vi "RunAllTests.vi"() -> ()   [LabVIEW 2019]
uses:
  <vilib>/Rock Robotics/WPI/ThirdParty/JAS_Junk/TrajLib/Trajectory_Library.lvlib
panel:
  out "Meca Drive \nPose Est 2":bool
  out "Swerve Module Position":bool
  out "Swerve Drive Pose Est 2":bool
  out "Diff Drive Pose Est 2":bool
  out "Diff Drive Odom 2":bool
  out "April Tag":bool
  out "Vector":bool
  out "Lead Lag":bool
  out "Elliptical Region\nConstraint":bool
  out "Rectangular Region\nConstraint":bool
  out "Meca Drive \nPose Est":bool
  out "Coordinate System":bool
  out "Meca Drive \nOdometry":bool
  out "Meca Drive \nKinematics":bool
  out "Pose3d":bool
  out "Transform3d":bool
  out "Rotation3d":bool
  out "Translation3d":bool
  out "Twist3d":bool
  out "Function Generator \nMatrix":bool
  out "LTV Unicycle \nController":bool
  out "LTV Diff Drive \nController":bool
  out "Time Interpolatable \nRotation2d":bool
  out "Time Interpolatable \nDouble":bool
  out "Time Interpolatable \nBoolean":bool
  out "Time Interpolatable \nPose2d":bool
  out "Implicit Model \nFollower":bool
  out "Function Generator":bool
  out "Diff Drive Accel Limiter":bool
  out "String":string
  out "Vision Utilities":bool
  out "Flywheel Simulation":bool
  out "DC Motor Simulation":bool
  out "Matrix":bool
  out "PID":bool
  out "Profiled PID \nInput/Output":bool
  out "Bang Bang \nInput/Output":bool
  out "Bang Bang Tolerance":bool
  out "Debounce":bool
  out "Math Utils":bool
  out "Linear Filter":bool
  out "State Space Util":bool
  out "Runge Kutta \nTime Varying":bool
  out "Linear System Loop":bool
  out "Swerve Drive \nKinematics":bool
  out "Swerve Drive Odometry":bool
  out "Trajectory Generate":bool
  out "Trajectory Transform":bool
  out "Units":bool
  out "All Tests Finished":bool
  out "Trajectory Concatenate":bool
  out "Trajectory JSON":bool
  out "Diff Drive Train Sim":bool
  out "Timer":bool
  out "Single Jointed \nArm Sim":bool
  out "Elevator Sim":bool
  out "Simple Motor \nFeedforward":bool
  out "Diff Drive Voltage \nConstraint":bool
  out "Diff Drive Pose Est":bool
  out "Holonomic Drive Ctrl":bool
  out "Linear Plant Inv FF":bool
  out "Centrip Accel \nConstraint":bool
  out "Diff Drive Kine \nConstraint":bool
  out "Controller Utility":bool
  out "Swerve Drive Pose Est":bool
  out "Swerve Module State":bool
  out "Trapezoid Profile":bool
  out "Slew Rate Limiter":bool
  out "Chassis Speeds":bool
  out "Numerical Jacobian":bool
  out "Merwe Scaled \nSigma Pts":bool
  out "Numerical Integration":bool
  out "DARE - Ricatti":bool
  out "Quintic Spline":bool
  out "Unscented Kalman \nFilter":bool
  out "Ramsete":bool
  out "Profiled PID":bool
  out "Twist":bool
  out "Translation2d":bool
  out "Transform2d":bool
  out "Rotation2d":bool
  out "Pose2d":bool
  out "Median Filter":bool
  out "Cubic Spline":bool
  out "Linear System ID":bool
  out "Kalman filter":bool
  out "Discretization":bool
  out "PID tolerance":bool
  out "PID Input / Output":bool
  out "Linear Quadradtic \nRegulator":bool
  out "Diff Drive Kinematics":bool
  out "Angle Stats":bool
  # "FORMAL TRAJECTORY / CONTROL LIBRARY TEST PROCEDURE"
  # "FUNCTION NOT\nIMPLEMENTED"
  # "Extended Kalman \nFilter"
  # "Cntrl Affine Plant \nInversion"
  # "FUNCTION NOT\nIMPLEMENTED"
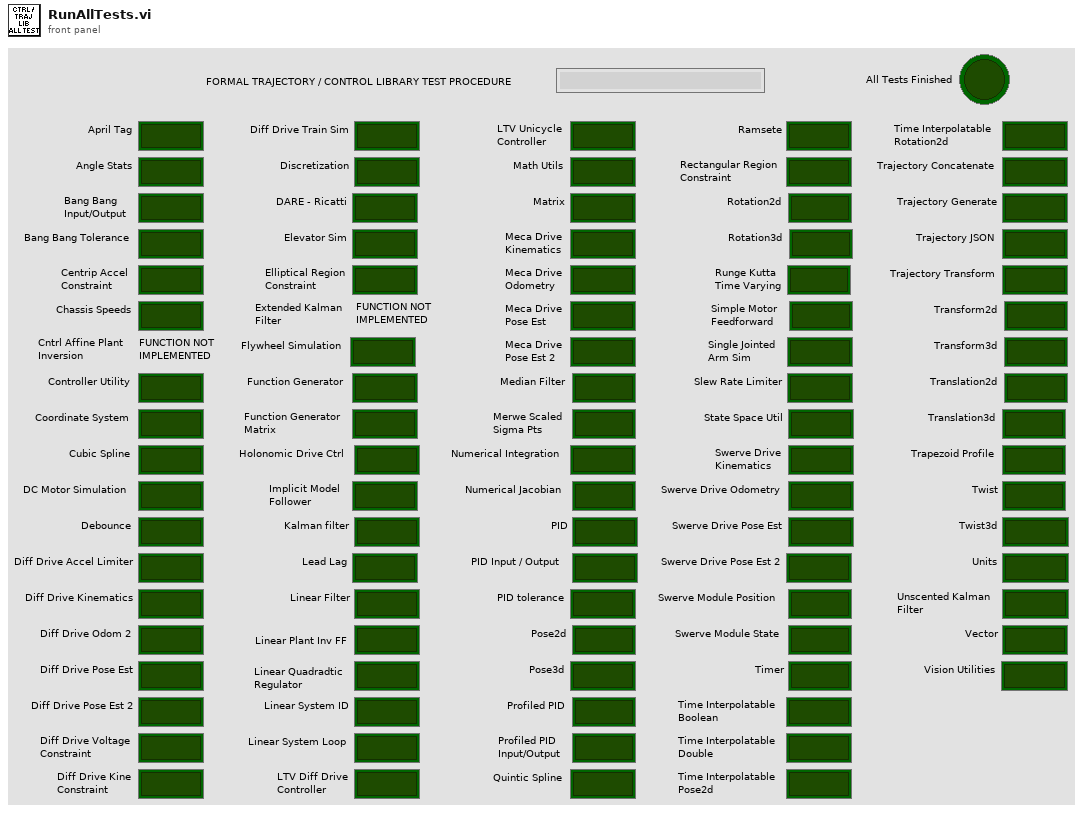
[diagram p1: front panel]
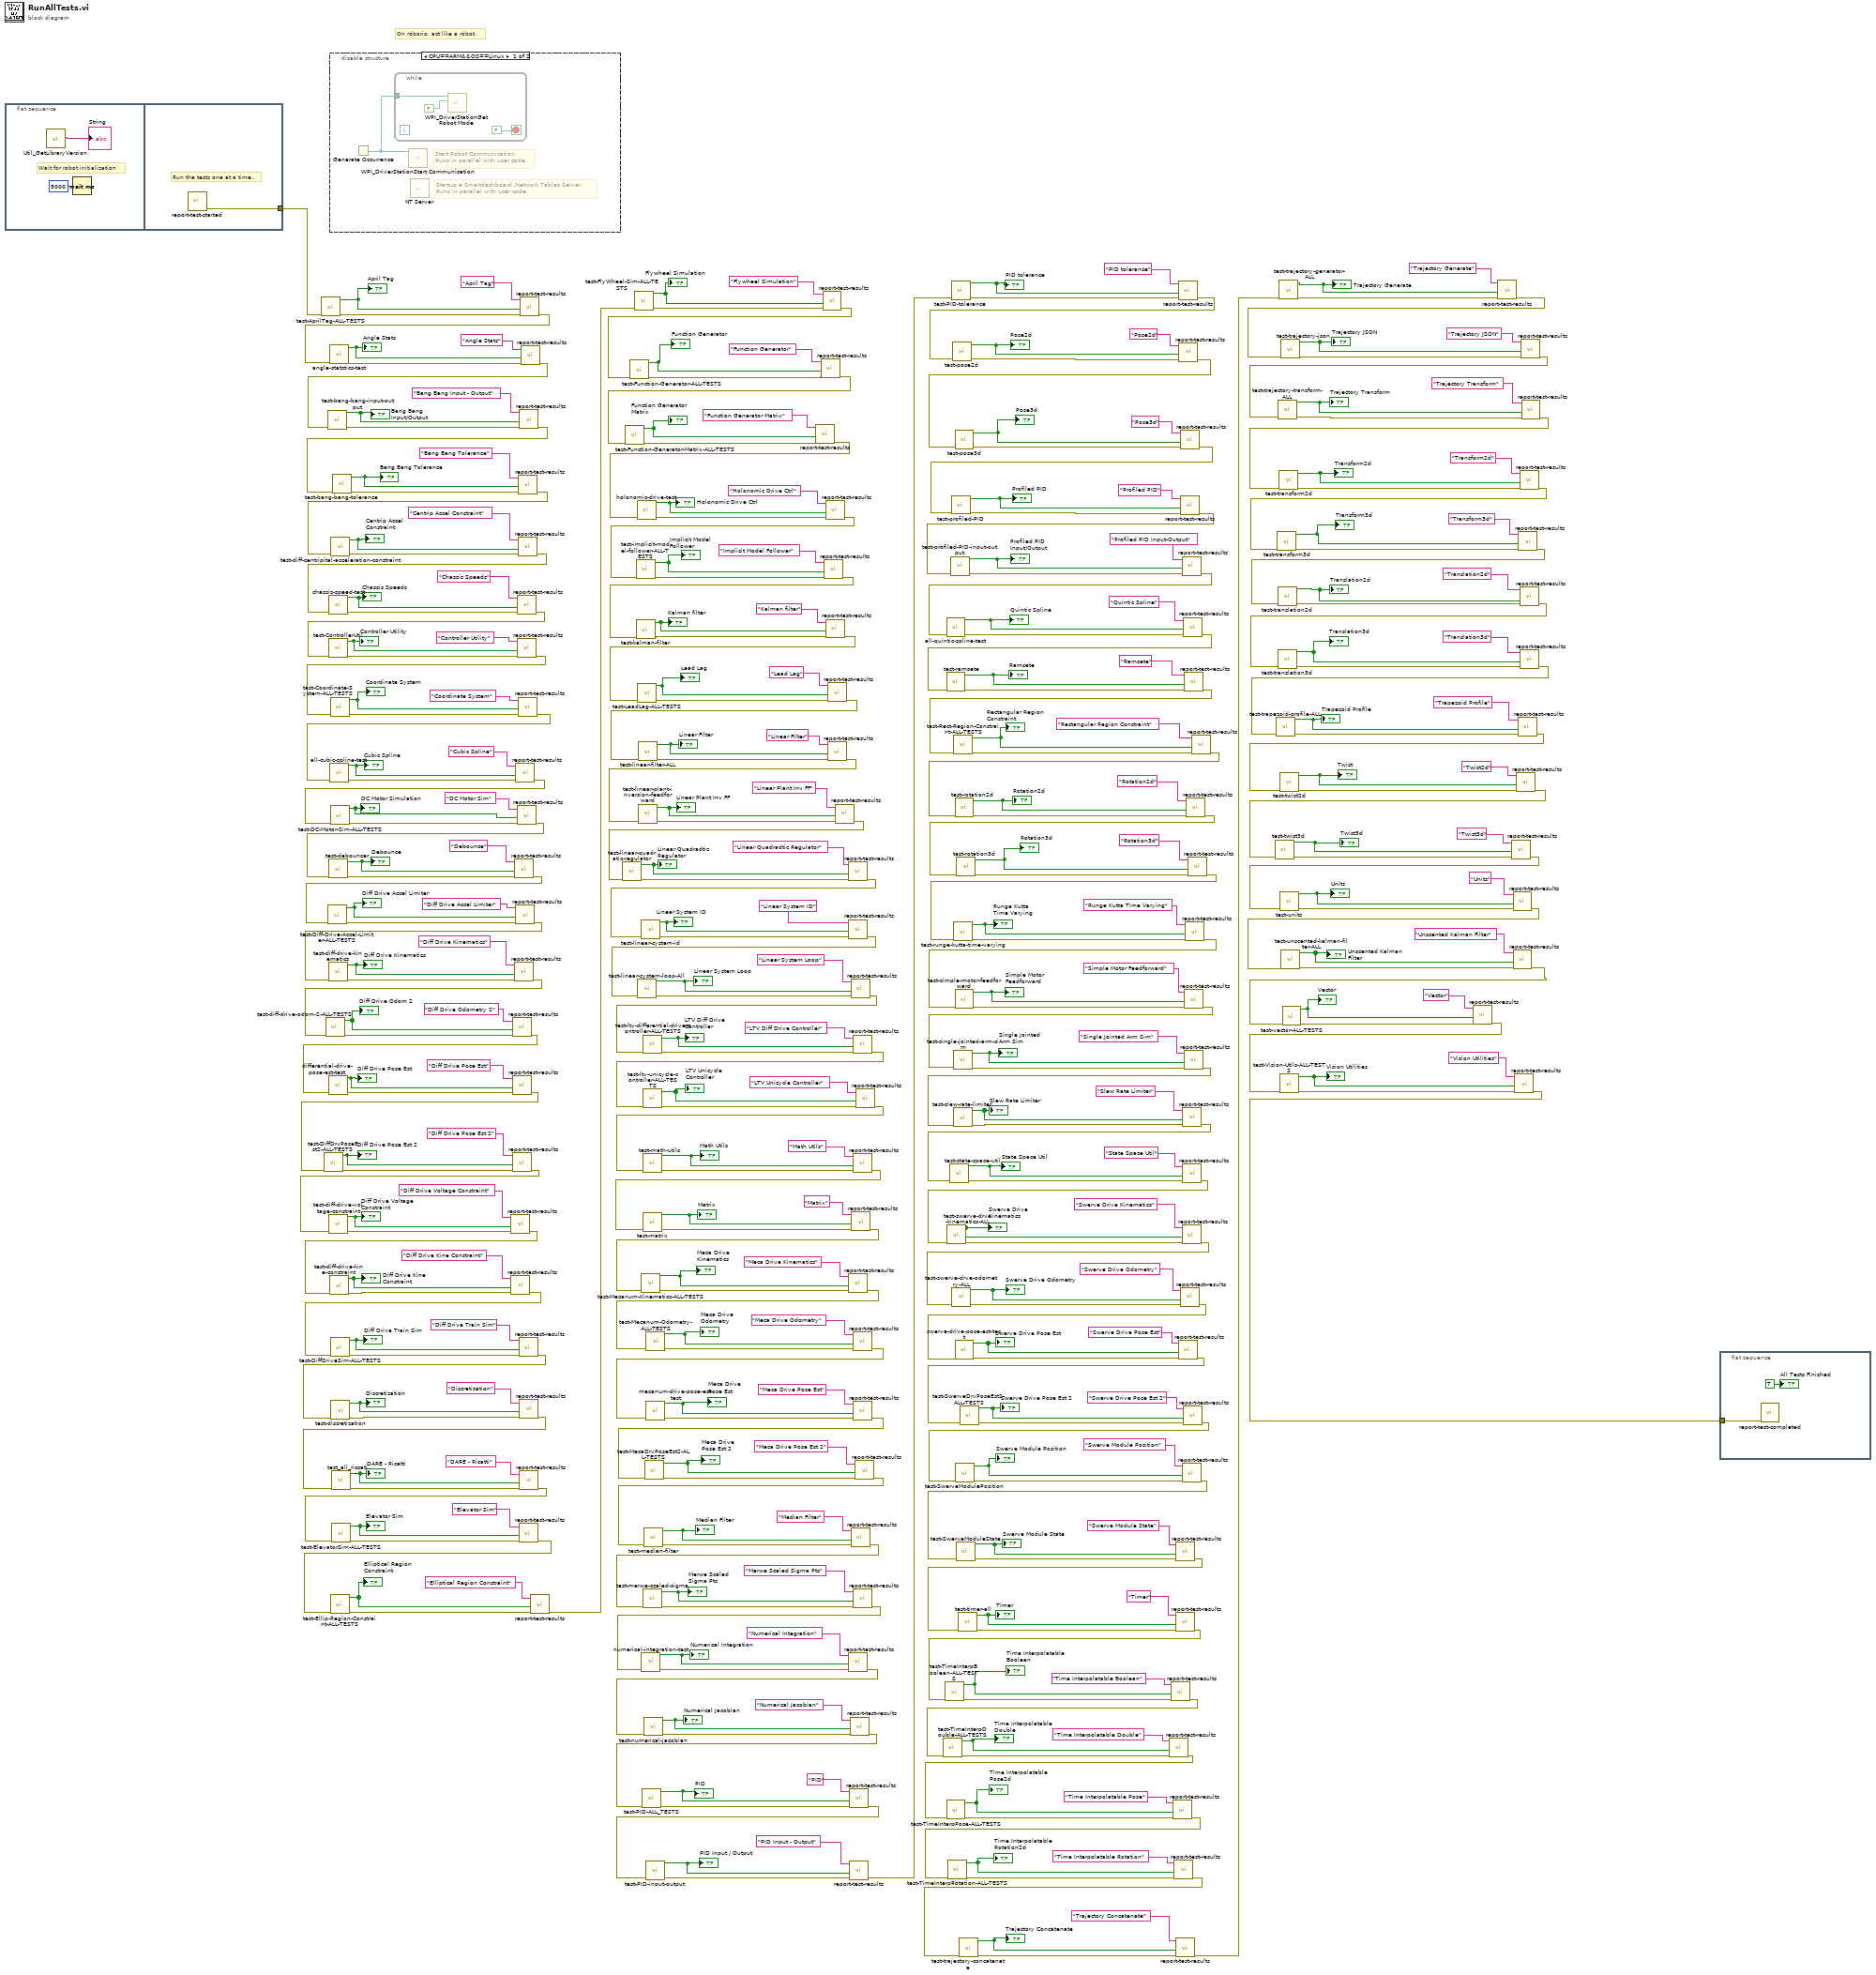
[diagram p0: block diagram]
diagram:
  # "On roborio, act like a robot."
  n1 = flat-sequence {
    tunnel: [w364] -> w16
    frame #0 {
      # "Wait for robot initialization"
      n2 = call <vilib>:"Util_GetLibraryVersion.vi"() -> ("TrajLibVersion"=→"String":string)  [unwired: 11 in]
      n3 = Wait (ms)(milliseconds to wait=u32 5000) -> ()  [unwired: 1 out]
    }
    frame #1 {
      # "Run the tests one at a time.."
      n4 = call "report-test-started.vi"() -> ("error out"=w364:errorcluster)  [unwired: 11 in]
    }
  }
  n5 = call "test-AprilTag-ALL-TESTS.vi"("error in (no error)"=w16) -> ("error out"=w29:errorcluster, "All Passed"=w28:bool)  [unwired: 9 in]
  "April Tag" <- w28
  n6 = disable-structure shown="CPU==ARM&&OS==Linux" {
    frame condition #0 {
      # "Startup a Smartdashboard /Network Tables Server.\nRuns in parallel with user code."
      # "Start Robot Communication.\nRuns in parallel with user code."
      n7 = Generate Occurrence() -> (w365:refnum<k4>)
      n8 = while {
        tunnel: w365 -> [w368]
        stop <- FALSE stop-if-true
        n9 = call <vilib>:"WPI_DriverStationGet Robot Mode.vi"("Finish"=FALSE, "DS Occurrence"=w368) -> ()  [unwired: 10 out]
      }
      n10 = call <vilib>:"WPI_DriverStationStart Communication.vi"("occurrence"=w365) -> ()  [unwired: 2 in, 9 out]
      n11 = call <vilib>:"NT Server.vi"() -> ()  [unwired: 11 in, 1 out]
    }
    frame condition #1 (active) {
    }
  }
  n12 = call "report-test-results.vi"("error in (no error)"=w29, "TestPassed"=w28, "Test Name"="April Tag") -> ("error out"=w15:errorcluster)  [unwired: 8 in]
  n13 = call "angle-statstics-test.vi"("error in (no error)"=w15) -> ("error out"=w244:errorcluster, "All Passed"=w361:bool)  [unwired: 9 in]
  "Angle Stats" <- w361
  n14 = call "report-test-results.vi"("error in (no error)"=w244, "TestPassed"=w361, "Test Name"="Angle Stats") -> ("error out"=w245:errorcluster)  [unwired: 8 in]
  n15 = call "test-bang-bang-input-output.vi"("error in (no error)"=w245) -> ("error out"=w243:errorcluster, "All Tests Passed"=w358:bool)  [unwired: 9 in]
  "Bang Bang \nInput/Output" <- w358
  n16 = call "report-test-results.vi"("error in (no error)"=w243, "TestPassed"=w358, "Test Name"="Bang Bang Input - Output") -> ("error out"=w242:errorcluster)  [unwired: 8 in]
  n17 = call "test-bang-bang-tolerance.vi"("error in (no error)"=w242) -> ("error out"=w241:errorcluster, "All Tests Passed"=w356:bool)  [unwired: 9 in]
  "Bang Bang Tolerance" <- w356
  n18 = call "report-test-results.vi"("error in (no error)"=w241, "TestPassed"=w356, "Test Name"="Bang Bang Tolerance") -> ("error out"=w240:errorcluster)  [unwired: 8 in]
  n19 = call "test-diff-centripital-acceleration-constraint.vi"("error in (no error)"=w240) -> ("error out 2"=w239:errorcluster, "Test Passed"=w354:bool)  [unwired: 9 in]
  "Centrip Accel \nConstraint" <- w354
  n20 = call "report-test-results.vi"("error in (no error)"=w239, "TestPassed"=w354, "Test Name"="Centrip Accel Constraint") -> ("error out"=w238:errorcluster)  [unwired: 8 in]
  n21 = call "chassis-speed-test.vi"("error in (no error)"=w238) -> ("error out"=w237:errorcluster, "Test Passed"=w352:bool)  [unwired: 9 in]
  "Chassis Speeds" <- w352
  n22 = call "report-test-results.vi"("error in (no error)"=w237, "TestPassed"=w352, "Test Name"="Chassis Speeds") -> ("error out"=w139:errorcluster)  [unwired: 8 in]
  n23 = call "test-ControllerUtil.vi"("error in (no error)"=w139) -> ("error out"=w236:errorcluster, "All Tests Passed"=w350:bool)  [unwired: 9 in]
  "Controller Utility" <- w350
  n24 = call "report-test-results.vi"("error in (no error)"=w236, "TestPassed"=w350, "Test Name"="Controller Utility") -> ("error out"=w58:errorcluster)  [unwired: 8 in]
  n25 = call "test-Coordinate-System-ALL-TESTS.vi"("error in (no error)"=w58) -> ("error out"=w59:errorcluster, "All Passed"=w56:bool)  [unwired: 9 in]
  "Coordinate System" <- w56
  n26 = call "report-test-results.vi"("error in (no error)"=w59, "TestPassed"=w56, "Test Name"="Coordinate System") -> ("error out"=w57:errorcluster)  [unwired: 8 in]
  n27 = call "all-cubic-spline-test.vi"("error in (no error)"=w57) -> ("error out"=w230:errorcluster, "ALL TESTS PASSED"=w346:bool)  [unwired: 9 in]
  "Cubic Spline" <- w346
  n28 = call "report-test-results.vi"("error in (no error)"=w230, "TestPassed"=w346, "Test Name"="Cubic Spline") -> ("error out"=w150:errorcluster)  [unwired: 8 in]
  n29 = call "test-DC-Motor-Sim-ALL-TESTS.vi"("error in (no error)"=w150) -> ("error out"=w148:errorcluster, "All Passed"=w147:bool)  [unwired: 9 in]
  "DC Motor Simulation" <- w147
  n30 = call "report-test-results.vi"("error in (no error)"=w148, "TestPassed"=w147, "Test Name"="DC Motor Sim") -> ("error out"=w146:errorcluster)  [unwired: 8 in]
  n31 = call "test-debouncer.vi"("error in (no error)"=w146) -> ("error out"=w229:errorcluster, "ALL TESTS PASSED"=w345:bool)  [unwired: 9 in]
  "Debounce" <- w345
  n32 = call "report-test-results.vi"("error in (no error)"=w229, "TestPassed"=w345, "Test Name"="Debounce") -> ("error out"=w136:errorcluster)  [unwired: 8 in]
  n33 = call "test-Diff-Drive-Accel-Limiter-ALL-TESTS.vi"("error in (no error)"=w136) -> ("error out"=w137:errorcluster, "All Passed"=w135:bool)  [unwired: 9 in]
  "Diff Drive Accel Limiter" <- w135
  n34 = call "report-test-results.vi"("error in (no error)"=w137, "TestPassed"=w135, "Test Name"="Diff Drive Accel Limiter") -> ("error out"=w134:errorcluster)  [unwired: 8 in]
  n35 = call "test-diff-drive-kinematics.vi"("error in (no error)"=w134) -> ("error out"=w228:errorcluster, "All Passed"=w344:bool)  [unwired: 9 in]
  "Diff Drive Kinematics" <- w344
  n36 = call "report-test-results.vi"("error in (no error)"=w228, "TestPassed"=w344, "Test Name"="Diff Drive Kinematics") -> ("error out"=w26:errorcluster)  [unwired: 8 in]
  n37 = call "test-diff-drive-odom-2-ALL-TESTS.vi"("error in (no error)"=w26) -> ("error out"=w25:errorcluster, "All Passed"=w24:bool)  [unwired: 9 in]
  "Diff Drive Odom 2" <- w24
  n38 = call "report-test-results.vi"("error in (no error)"=w25, "TestPassed"=w24, "Test Name"="Diff Drive Odometry 2") -> ("error out"=w23:errorcluster)  [unwired: 8 in]
  n39 = call "differential-drive-pose-est-test.vi"("error in (no error)"=w23) -> ("error out"=w227:errorcluster, "Test Passed"=w340:bool)  [unwired: 9 in]
  "Diff Drive Pose Est" <- w340
  n40 = call "report-test-results.vi"("error in (no error)"=w227, "TestPassed"=w340, "Test Name"="Diff Drive Pose Est") -> ("error out"=w21:errorcluster)  [unwired: 8 in]
  n41 = call "test-DiffDrvPoseEst2-ALL-TESTS.vi"("error in (no error)"=w21) -> ("error out"=w20:errorcluster, "All Passed"=w19:bool)  [unwired: 9 in]
  "Diff Drive Pose Est 2" <- w19
  n42 = call "report-test-results.vi"("error in (no error)"=w20, "TestPassed"=w19, "Test Name"="Diff Drive Pose Est 2") -> ("error out"=w18:errorcluster)  [unwired: 8 in]
  n43 = call "test-diff-drive-voltage-constraint.vi"("error in (no error)"=w18) -> ("error out 4"=w226:errorcluster, "Test Passed"=w339:bool)  [unwired: 9 in]
  "Diff Drive Voltage \nConstraint" <- w339
  n44 = call "report-test-results.vi"("error in (no error)"=w226, "TestPassed"=w339, "Test Name"="Diff Drive Voltage Constraint") -> ("error out"=w221:errorcluster)  [unwired: 8 in]
  n45 = call "test-diff-drive-kine-constraint.vi"("error in (no error)"=w221) -> ("error out 2"=w225:errorcluster, "Test Passed"=w338:bool)  [unwired: 9 in]
  "Diff Drive Kine \nConstraint" <- w338
  n46 = call "report-test-results.vi"("error in (no error)"=w225, "TestPassed"=w338, "Test Name"="Diff Drive Kine Constraint") -> ("error out"=w220:errorcluster)  [unwired: 8 in]
  n47 = call "test-DiffDriveSim-ALL-TESTS.vi"("error in (no error)"=w220) -> ("error out"=w224:errorcluster, "All Passed"=w334:bool)  [unwired: 9 in]
  "Diff Drive Train Sim" <- w334
  n48 = call "report-test-results.vi"("error in (no error)"=w224, "TestPassed"=w334, "Test Name"="Diff Drive Train Sim") -> ("error out"=w219:errorcluster)  [unwired: 8 in]
  n49 = call "test-discretization.vi"("error in (no error)"=w219) -> ("error out"=w223:errorcluster, "All Tests Passed"=w333:bool)  [unwired: 9 in]
  "Discretization" <- w333
  n50 = call "report-test-results.vi"("error in (no error)"=w223, "TestPassed"=w333, "Test Name"="Discretization") -> ("error out"=w218:errorcluster)  [unwired: 8 in]
  n51 = call "test_all_riccati.vi"("error in (no error)"=w218) -> ("error out"=w222:errorcluster, "All Tests Passed"=w332:bool)  [unwired: 9 in]
  "DARE - Ricatti" <- w332
  n52 = call "report-test-results.vi"("error in (no error)"=w222, "TestPassed"=w332, "Test Name"="DARE - Ricatti") -> ("error out"=w43:errorcluster)  [unwired: 8 in]
  n53 = call "test-ElevatorSim-ALL-TESTS.vi"("error in (no error)"=w43) -> ("error out"=w235:errorcluster, "All Passed"=w328:bool)  [unwired: 9 in]
  "Elevator Sim" <- w328
  n54 = call "report-test-results.vi"("error in (no error)"=w235, "TestPassed"=w328, "Test Name"="Elevator Sim") -> ("error out"=w41:errorcluster)  [unwired: 8 in]
  n55 = call "test-Ellip-Region-Constraint-ALL-TESTS.vi"("error in (no error)"=w41) -> ("error out"=w45:errorcluster, "All Passed"=w44:bool)  [unwired: 9 in]
  "Elliptical Region\nConstraint" <- w44
  n56 = call "report-test-results.vi"("error in (no error)"=w45, "TestPassed"=w44, "Test Name"="Elliptical Region Constraint") -> ("error out"=w42:errorcluster)  [unwired: 8 in]
  n57 = call "test-FlyWheel-Sim-ALL-TESTS.vi"("error in (no error)"=w42) -> ("error out"=w144:errorcluster, "All Passed"=w143:bool)  [unwired: 9 in]
  "Flywheel Simulation" <- w143
  n58 = call "report-test-results.vi"("error in (no error)"=w144, "TestPassed"=w143, "Test Name"="Flywheel Simulation") -> ("error out"=w132:errorcluster)  [unwired: 8 in]
  n59 = call "test-Function-Generator-ALL-TESTS.vi"("error in (no error)"=w132) -> ("error out"=w130:errorcluster, "All Passed"=w131:bool)  [unwired: 9 in]
  "Function Generator" <- w131
  n60 = call "report-test-results.vi"("error in (no error)"=w130, "TestPassed"=w131, "Test Name"="Function Generator") -> ("error out"=w95:errorcluster)  [unwired: 8 in]
  n61 = call "test-Function-Generator-Matrix-ALL-TESTS.vi"("error in (no error)"=w95) -> ("error out"=w97:errorcluster, "All Passed"=w96:bool)  [unwired: 9 in]
  "Function Generator \nMatrix" <- w96
  n62 = call "report-test-results.vi"("error in (no error)"=w97, "TestPassed"=w96, "Test Name"="Function Generator Matrix") -> ("error out"=w94:errorcluster)  [unwired: 8 in]
  n63 = call "holonomic-drive-test.vi"("error in (no error)"=w94) -> ("error out"=w234:errorcluster, "ALL TESTS PASSED"=w327:bool)  [unwired: 9 in]
  "Holonomic Drive Ctrl" <- w327
  n64 = call "report-test-results.vi"("error in (no error)"=w234, "TestPassed"=w327, "Test Name"="Holonomic Drive Ctrl") -> ("error out"=w126:errorcluster)  [unwired: 8 in]
  n65 = call "test-implicit-model-follower-ALL-TESTS.vi"("error in (no error)"=w126) -> ("error out"=w128:errorcluster, "All Passed"=w125:bool)  [unwired: 9 in]
  "Implicit Model \nFollower" <- w125
  n66 = call "report-test-results.vi"("error in (no error)"=w128, "TestPassed"=w125, "Test Name"="Implicit Model Follower") -> ("error out"=w127:errorcluster)  [unwired: 8 in]
  n67 = call "test-kalman-filter.vi"("error in (no error)"=w127) -> ("error out"=w233:errorcluster, "ALL TESTS PASSED"=w326:bool)  [unwired: 9 in]
  "Kalman filter" <- w326
  n68 = call "report-test-results.vi"("error in (no error)"=w233, "TestPassed"=w326, "Test Name"="Kalman filter") -> ("error out"=w38:errorcluster)  [unwired: 8 in]
  n69 = call "test-LeadLag-ALL-TESTS.vi"("error in (no error)"=w38) -> ("error out"=w39:errorcluster, "All Passed"=w36:bool)  [unwired: 9 in]
  "Lead Lag" <- w36
  n70 = call "report-test-results.vi"("error in (no error)"=w39, "TestPassed"=w36, "Test Name"="Lead Lag") -> ("error out"=w37:errorcluster)  [unwired: 8 in]
  n71 = call "test-linear-filter-ALL.vi"("error in (no error)"=w37) -> ("error out"=w217:errorcluster, "ALL TESTS GOOD"=w317:bool)  [unwired: 9 in]
  "Linear Filter" <- w317
  n72 = call "report-test-results.vi"("error in (no error)"=w217, "TestPassed"=w317, "Test Name"="Linear Filter") -> ("error out"=w216:errorcluster)  [unwired: 8 in]
  n73 = call "test-linear-plant-inversion-feedforward.vi"("error in (no error)"=w216) -> ("error out"=w215:errorcluster, "All Tests Passed"=w316:bool)  [unwired: 9 in]
  "Linear Plant Inv FF" <- w316
  n74 = call "report-test-results.vi"("error in (no error)"=w215, "TestPassed"=w316, "Test Name"="Linear Plant Inv FF") -> ("error out"=w214:errorcluster)  [unwired: 8 in]
  n75 = call "test-linear-quadratic-regulator.vi"("error in (no error)"=w214) -> ("error out"=w213:errorcluster, "ALL TESTS GOOD"=w315:bool)  [unwired: 9 in]
  "Linear Quadradtic \nRegulator" <- w315
  n76 = call "report-test-results.vi"("error in (no error)"=w213, "TestPassed"=w315, "Test Name"="Linear Quadradtic Regulator") -> ("error out"=w212:errorcluster)  [unwired: 8 in]
  n77 = call "test-linear-system-id.vi"("error in (no error)"=w212) -> ("error out"=w211:errorcluster, "All tests passed"=w314:bool)  [unwired: 9 in]
  "Linear System ID" <- w314
  n78 = call "report-test-results.vi"("error in (no error)"=w211, "TestPassed"=w314, "Test Name"="Linear System ID") -> ("error out"=w203:errorcluster)  [unwired: 8 in]
  n79 = call "test-linear-system-loop-All.vi"("error in (no error)"=w203) -> ("error out"=w204:errorcluster, "ALL TEsts Passed"=w313:bool)  [unwired: 9 in]
  "Linear System Loop" <- w313
  n80 = call "report-test-results.vi"("error in (no error)"=w204, "TestPassed"=w313, "Test Name"="Linear System Loop") -> ("error out"=w103:errorcluster)  [unwired: 8 in]
  n81 = call "test-ltv-differential-drive-controller-ALL-TESTS.vi"("error in (no error)"=w103) -> ("error out"=w104:errorcluster, "All Passed"=w105:bool)  [unwired: 9 in]
  "LTV Diff Drive \nController" <- w105
  n82 = call "report-test-results.vi"("error in (no error)"=w104, "TestPassed"=w105, "Test Name"="LTV Diff Drive Controller") -> ("error out"=w100:errorcluster)  [unwired: 8 in]
  n83 = call "test-ltv-unicycle-controller-ALL-TESTS.vi"("error in (no error)"=w100) -> ("error out"=w102:errorcluster, "All Passed"=w101:bool)  [unwired: 9 in]
  "LTV Unicycle \nController" <- w101
  n84 = call "report-test-results.vi"("error in (no error)"=w102, "TestPassed"=w101, "Test Name"="LTV Unicycle Controller") -> ("error out"=w99:errorcluster)  [unwired: 8 in]
  n85 = call "test-math-utils.vi"("error in (no error)"=w99) -> ("error out"=w202:errorcluster, "ALL TESTS PASSED"=w312:bool)  [unwired: 9 in]
  "Math Utils" <- w312
  n86 = call "report-test-results.vi"("error in (no error)"=w202, "TestPassed"=w312, "Test Name"="Math Utils") -> ("error out"=w201:errorcluster)  [unwired: 8 in]
  n87 = call "test-matrix.vi"("error in (no error)"=w201) -> ("error out"=w205:errorcluster, "All Tests\nPassed"=w311:bool)  [unwired: 9 in]
  "Matrix" <- w311
  n88 = call "report-test-results.vi"("error in (no error)"=w205, "TestPassed"=w311, "Test Name"="Matrix") -> ("error out"=w65:errorcluster)  [unwired: 8 in]
  n89 = call "test-Mecanum-Kinematics-ALL-TESTS.vi"("error in (no error)"=w65) -> ("error out"=w67:errorcluster, "All Passed"=w66:bool)  [unwired: 9 in]
  "Meca Drive \nKinematics" <- w66
  n90 = call "report-test-results.vi"("error in (no error)"=w67, "TestPassed"=w66, "Test Name"="Meca Drive Kinematics") -> ("error out"=w62:errorcluster)  [unwired: 8 in]
  n91 = call "test-Mecanum-Odometry-ALL-TESTS.vi"("error in (no error)"=w62) -> ("error out"=w63:errorcluster, "All Passed"=w61:bool)  [unwired: 9 in]
  "Meca Drive \nOdometry" <- w61
  n92 = call "report-test-results.vi"("error in (no error)"=w63, "TestPassed"=w61, "Test Name"="Meca Drive Odometry") -> ("error out"=w52:errorcluster)  [unwired: 8 in]
  n93 = call "mecanum-drive-pose-est-test.vi"("error in (no error)"=w52) -> ("error out"=w54:errorcluster, "Test Passed"=w53:bool)  [unwired: 9 in]
  "Meca Drive \nPose Est" <- w53
  n94 = call "report-test-results.vi"("error in (no error)"=w54, "TestPassed"=w53, "Test Name"="Meca Drive Pose Est") -> ("error out"=w4:errorcluster)  [unwired: 8 in]
  n95 = call "test-MecaDrvPoseEst2-ALL-TESTS.vi"("error in (no error)"=w4) -> ("error out"=w3:errorcluster, "All Passed"=w2:bool)  [unwired: 9 in]
  "Meca Drive \nPose Est 2" <- w2
  n96 = call "report-test-results.vi"("error in (no error)"=w3, "TestPassed"=w2, "Test Name"="Meca Drive Pose Est 2") -> ("error out"=w1:errorcluster)  [unwired: 8 in]
  n97 = call "test-median-filter.vi"("error in (no error)"=w1) -> ("error out"=w206:errorcluster, "ALL TESTS PASSED"=w310:bool)  [unwired: 9 in]
  "Median Filter" <- w310
  n98 = call "report-test-results.vi"("error in (no error)"=w206, "TestPassed"=w310, "Test Name"="Median Filter") -> ("error out"=w200:errorcluster)  [unwired: 8 in]
  n99 = call "test-merwe-scaled-sigma.vi"("error in (no error)"=w200) -> ("error out"=w207:errorcluster, "All Tests Passed"=w296:bool)  [unwired: 9 in]
  "Merwe Scaled \nSigma Pts" <- w296
  n100 = call "report-test-results.vi"("error in (no error)"=w207, "TestPassed"=w296, "Test Name"="Merwe Scaled Sigma Pts") -> ("error out"=w199:errorcluster)  [unwired: 8 in]
  n101 = call "numerical-integration-test.vi"("error in (no error)"=w199) -> ("error out"=w208:errorcluster, "All passed"=w297:bool)  [unwired: 9 in]
  "Numerical Integration" <- w297
  n102 = call "report-test-results.vi"("error in (no error)"=w208, "TestPassed"=w297, "Test Name"="Numerical Integration") -> ("error out"=w198:errorcluster)  [unwired: 8 in]
  n103 = call "test-numerical-jacobian.vi"("error in (no error)"=w198) -> ("error out"=w209:errorcluster, "ALL Tests Passed"=w298:bool)  [unwired: 9 in]
  "Numerical Jacobian" <- w298
  n104 = call "report-test-results.vi"("error in (no error)"=w209, "TestPassed"=w298, "Test Name"="Numerical Jacobian") -> ("error out"=w197:errorcluster)  [unwired: 8 in]
  n105 = call "test-PID-ALL_TESTS.vi"("error in (no error)"=w197) -> ("error out"=w210:errorcluster, "All Passed"=w299:bool)  [unwired: 9 in]
  "PID" <- w299
  n106 = call "report-test-results.vi"("error in (no error)"=w210, "TestPassed"=w299, "Test Name"="PID") -> ("error out"=w196:errorcluster)  [unwired: 8 in]
  n107 = call "test-PID-input-output.vi"("error in (no error)"=w196) -> ("error out"=w231:errorcluster, "All Passed"=w300:bool)  [unwired: 9 in]
  "PID Input / Output" <- w300
  n108 = call "report-test-results.vi"("error in (no error)"=w231, "TestPassed"=w300, "Test Name"="PID Input - Output") -> ("error out"=w232:errorcluster)  [unwired: 8 in]
  n109 = call "test-PID-tolerance.vi"("error in (no error)"=w232) -> ("error out"=w194:errorcluster, "All Tests Passed"=w301:bool)  [unwired: 9 in]
  "PID tolerance" <- w301
  n110 = call "report-test-results.vi"("error in (no error)"=w194, "TestPassed"=w301, "Test Name"="PID tolerance") -> ("error out"=w177:errorcluster)  [unwired: 8 in]
  n111 = call "test-pose2d.vi"("error in (no error)"=w177) -> ("error out"=w193:errorcluster, "All PASSED"=w302:bool)  [unwired: 9 in]
  "Pose2d" <- w302
  n112 = call "report-test-results.vi"("error in (no error)"=w193, "TestPassed"=w302, "Test Name"="Pose2d") -> ("error out"=w71:errorcluster)  [unwired: 8 in]
  n113 = call "test-pose3d.vi"("error in (no error)"=w71) -> ("error out"=w72:errorcluster, "All PASSED"=w69:bool)  [unwired: 9 in]
  "Pose3d" <- w69
  n114 = call "report-test-results.vi"("error in (no error)"=w72, "TestPassed"=w69, "Test Name"="Pose3d") -> ("error out"=w70:errorcluster)  [unwired: 8 in]
  n115 = call "test-profiled-PID.vi"("error in (no error)"=w70) -> ("error out"=w192:errorcluster, "Test Passed 0"=w284:bool)  [unwired: 9 in]
  "Profiled PID" <- w284
  n116 = call "report-test-results.vi"("error in (no error)"=w192, "TestPassed"=w284, "Test Name"="Profiled PID") -> ("error out"=w176:errorcluster)  [unwired: 8 in]
  n117 = call "test-profiled-PID-input-output.vi"("error in (no error)"=w176) -> ("error out"=w191:errorcluster, "All Tests Passed"=w283:bool)  [unwired: 9 in]
  "Profiled PID \nInput/Output" <- w283
  n118 = call "report-test-results.vi"("error in (no error)"=w191, "TestPassed"=w283, "Test Name"="Profiled PID Input-Output") -> ("error out"=w175:errorcluster)  [unwired: 8 in]
  n119 = call "all-quintic-spline-test.vi"("error in (no error)"=w175) -> ("error out"=w190:errorcluster, "ALL TESTS PASSED"=w282:bool)  [unwired: 9 in]
  "Quintic Spline" <- w282
  n120 = call "report-test-results.vi"("error in (no error)"=w190, "TestPassed"=w282, "Test Name"="Quintic Spline") -> ("error out"=w174:errorcluster)  [unwired: 8 in]
  n121 = call "test-ramsete.vi"("error in (no error)"=w174) -> ("error out"=w178:errorcluster, "AtReference End"=w281:bool)  [unwired: 9 in]
  "Ramsete" <- w281
  n122 = call "report-test-results.vi"("error in (no error)"=w178, "TestPassed"=w281, "Test Name"="Ramsete") -> ("error out"=w49:errorcluster)  [unwired: 8 in]
  n123 = call "test-Rect-Region-Constraint-ALL-TESTS.vi"("error in (no error)"=w49) -> ("error out"=w50:errorcluster, "All Passed"=w47:bool)  [unwired: 9 in]
  "Rectangular Region\nConstraint" <- w47
  n124 = call "report-test-results.vi"("error in (no error)"=w50, "TestPassed"=w47, "Test Name"="Rectangular Region Constraint") -> ("error out"=w48:errorcluster)  [unwired: 8 in]
  n125 = call "test-rotation2d.vi"("error in (no error)"=w48) -> ("error out"=w179:errorcluster, "ALL TESTS PASSED"=w280:bool)  [unwired: 9 in]
  "Rotation2d" <- w280
  n126 = call "report-test-results.vi"("error in (no error)"=w179, "TestPassed"=w280, "Test Name"="Rotation2d") -> ("error out"=w81:errorcluster)  [unwired: 8 in]
  n127 = call "test-rotation3d.vi"("error in (no error)"=w81) -> ("error out"=w82:errorcluster, "ALL TESTS PASSED"=w79:bool)  [unwired: 9 in]
  "Rotation3d" <- w79
  n128 = call "report-test-results.vi"("error in (no error)"=w82, "TestPassed"=w79, "Test Name"="Rotation3d") -> ("error out"=w80:errorcluster)  [unwired: 8 in]
  n129 = call "test-runge-kutta-time-varying.vi"("error in (no error)"=w80) -> ("error out"=w180:errorcluster, "Test Passed"=w279:bool)  [unwired: 9 in]
  "Runge Kutta \nTime Varying" <- w279
  n130 = call "report-test-results.vi"("error in (no error)"=w180, "TestPassed"=w279, "Test Name"="Runge Kutta Time Varying") -> ("error out"=w173:errorcluster)  [unwired: 8 in]
  n131 = call "test-simple-motor-feedforward.vi"("error in (no error)"=w173) -> ("error out"=w181:errorcluster, "All Tests Passed"=w278:bool)  [unwired: 9 in]
  "Simple Motor \nFeedforward" <- w278
  n132 = call "report-test-results.vi"("error in (no error)"=w181, "TestPassed"=w278, "Test Name"="Simple Motor Feedforward") -> ("error out"=w172:errorcluster)  [unwired: 8 in]
  n133 = call "test-single-jointed-arm-sim.vi"("error in (no error)"=w172) -> ("error out"=w182:errorcluster, "Test Passed"=w277:bool)  [unwired: 9 in]
  "Single Jointed \nArm Sim" <- w277
  n134 = call "report-test-results.vi"("error in (no error)"=w182, "TestPassed"=w277, "Test Name"="Single Jointed Arm Sim") -> ("error out"=w171:errorcluster)  [unwired: 8 in]
  n135 = call "test-slew-rate-limiter.vi"("error in (no error)"=w171) -> ("error out"=w183:errorcluster, "All Tests Passed"=w276:bool)  [unwired: 9 in]
  "Slew Rate Limiter" <- w276
  n136 = call "report-test-results.vi"("error in (no error)"=w183, "TestPassed"=w276, "Test Name"="Slew Rate Limiter") -> ("error out"=w170:errorcluster)  [unwired: 8 in]
  n137 = call "test-state-space-util.vi"("error in (no error)"=w170) -> ("error out"=w184:errorcluster, "All Tests Passed"=w275:bool)  [unwired: 9 in]
  "State Space Util" <- w275
  n138 = call "report-test-results.vi"("error in (no error)"=w184, "TestPassed"=w275, "Test Name"="State Space Util") -> ("error out"=w169:errorcluster)  [unwired: 8 in]
  n139 = call "test-swerve-drve-kinematics-ALL.vi"("error in (no error)"=w169) -> ("error out"=w185:errorcluster, "ALL TEsts Passed"=w274:bool)  [unwired: 9 in]
  "Swerve Drive \nKinematics" <- w274
  n140 = call "report-test-results.vi"("error in (no error)"=w185, "TestPassed"=w274, "Test Name"="Swerve Drive Kinematics") -> ("error out"=w168:errorcluster)  [unwired: 8 in]
  n141 = call "test-swerve-drve-odometry-ALL.vi"("error in (no error)"=w168) -> ("error out"=w186:errorcluster, "ALL TEsts Passed"=w271:bool)  [unwired: 9 in]
  "Swerve Drive Odometry" <- w271
  n142 = call "report-test-results.vi"("error in (no error)"=w186, "TestPassed"=w271, "Test Name"="Swerve Drive Odometry") -> ("error out"=w167:errorcluster)  [unwired: 8 in]
  n143 = call "swerve-drive-pose-est-test.vi"("error in (no error)"=w167) -> ("error out"=w187:errorcluster, "Test Passed"=w270:bool)  [unwired: 9 in]
  "Swerve Drive Pose Est" <- w270
  n144 = call "report-test-results.vi"("error in (no error)"=w187, "TestPassed"=w270, "Test Name"="Swerve Drive Pose Est") -> ("error out"=w11:errorcluster)  [unwired: 8 in]
  n145 = call "test-SwerveDrvPoseEst2-ALL-TESTS.vi"("error in (no error)"=w11) -> ("error out"=w12:errorcluster, "All Passed"=w13:bool)  [unwired: 9 in]
  "Swerve Drive Pose Est 2" <- w13
  n146 = call "report-test-results.vi"("error in (no error)"=w12, "TestPassed"=w13, "Test Name"="Swerve Drive Pose Est 2") -> ("error out"=w7:errorcluster)  [unwired: 8 in]
  n147 = call "test-SwerveModulePosition.vi"("error in (no error)"=w7) -> ("error out"=w9:errorcluster, "ALL TESTS PASSED"=w8:bool)  [unwired: 9 in]
  "Swerve Module Position" <- w8
  n148 = call "report-test-results.vi"("error in (no error)"=w9, "TestPassed"=w8, "Test Name"="Swerve Module Position") -> ("error out"=w6:errorcluster)  [unwired: 8 in]
  n149 = call "test-SwerveModuleState.vi"("error in (no error)"=w6) -> ("error out"=w188:errorcluster, "ALL TESTS PASSED"=w265:bool)  [unwired: 9 in]
  "Swerve Module State" <- w265
  n150 = call "report-test-results.vi"("error in (no error)"=w188, "TestPassed"=w265, "Test Name"="Swerve Module State") -> ("error out"=w166:errorcluster)  [unwired: 8 in]
  n151 = call "test-timer-all.vi"("error in (no error)"=w166) -> ("error out"=w165:errorcluster, "ALL TESTS PASSED"=w264:bool)  [unwired: 9 in]
  "Timer" <- w264
  n152 = call "report-test-results.vi"("error in (no error)"=w165, "TestPassed"=w264, "Test Name"="Timer") -> ("error out"=w115:errorcluster)  [unwired: 8 in]
  n153 = call "test-TimeInterpBoolean-ALL-TESTS.vi"("error in (no error)"=w115) -> ("error out"=w120:errorcluster, "All Passed"=w117:bool)  [unwired: 9 in]
  "Time Interpolatable \nBoolean" <- w117
  n154 = call "report-test-results.vi"("error in (no error)"=w120, "TestPassed"=w117, "Test Name"="Time Interpolatable Boolean") -> ("error out"=w114:errorcluster)  [unwired: 8 in]
  n155 = call "test-TimeInterpDouble-ALL-TESTS.vi"("error in (no error)"=w114) -> ("error out"=w118:errorcluster, "All Passed"=w116:bool)  [unwired: 9 in]
  "Time Interpolatable \nDouble" <- w116
  n156 = call "report-test-results.vi"("error in (no error)"=w118, "TestPassed"=w116, "Test Name"="Time Interpolatable Double") -> ("error out"=w113:errorcluster)  [unwired: 8 in]
  n157 = call "test-TimeInterpPose-ALL-TESTS.vi"("error in (no error)"=w113) -> ("error out"=w123:errorcluster, "All Passed"=w122:bool)  [unwired: 9 in]
  "Time Interpolatable \nPose2d" <- w122
  n158 = call "report-test-results.vi"("error in (no error)"=w123, "TestPassed"=w122, "Test Name"="Time Interpolatable Pose") -> ("error out"=w110:errorcluster)  [unwired: 8 in]
  n159 = call "test-TimeInterpRotation-ALL-TESTS.vi"("error in (no error)"=w110) -> ("error out"=w111:errorcluster, "All Passed"=w108:bool)  [unwired: 9 in]
  "Time Interpolatable \nRotation2d" <- w108
  n160 = call "report-test-results.vi"("error in (no error)"=w111, "TestPassed"=w108, "Test Name"="Time Interpolatable Rotation") -> ("error out"=w109:errorcluster)  [unwired: 8 in]
  n161 = call "test-trajectory-concatenate.vi"("error in (no error)"=w109) -> ("error out"=w189:errorcluster, "TEsts Passed"=w263:bool)  [unwired: 9 in]
  "Trajectory Concatenate" <- w263
  n162 = call "report-test-results.vi"("error in (no error)"=w189, "TestPassed"=w263, "Test Name"="Trajectory Concatenate") -> ("error out"=w152:errorcluster)  [unwired: 8 in]
  n163 = call "test-trajectory-generator-ALL.vi"("error in (no error)"=w152) -> ("error out"=w195:errorcluster, "ALL TESTS PASSED"=w262:bool)  [unwired: 9 in]
  "Trajectory Generate" <- w262
  n164 = call "report-test-results.vi"("error in (no error)"=w195, "TestPassed"=w262, "Test Name"="Trajectory Generate") -> ("error out"=w151:errorcluster)  [unwired: 8 in]
  n165 = call "test-trajectory-json.vi"("error in (no error)"=w151) -> ("error out 2"=w159:errorcluster, "ALL TESTS PASSED"=w254:bool)  [unwired: 9 in]
  "Trajectory JSON" <- w254
  n166 = call "report-test-results.vi"("error in (no error)"=w159, "TestPassed"=w254, "Test Name"="Trajectory JSON") -> ("error out"=w155:errorcluster)  [unwired: 8 in]
  n167 = call "test-trajectory-transform-ALL.vi"("error in (no error)"=w155) -> ("error out 2"=w158:errorcluster, "Test Passed"=w253:bool)  [unwired: 9 in]
  "Trajectory Transform" <- w253
  n168 = call "report-test-results.vi"("error in (no error)"=w158, "TestPassed"=w253, "Test Name"="Trajectory Transform") -> ("error out"=w154:errorcluster)  [unwired: 8 in]
  n169 = call "test-transform2d.vi"("error in (no error)"=w154) -> ("error out"=w160:errorcluster, "All PASSED"=w252:bool)  [unwired: 9 in]
  "Transform2d" <- w252
  n170 = call "report-test-results.vi"("error in (no error)"=w160, "TestPassed"=w252, "Test Name"="Transform2d") -> ("error out"=w76:errorcluster)  [unwired: 8 in]
  n171 = call "test-transform3d.vi"("error in (no error)"=w76) -> ("error out"=w77:errorcluster, "All PASSED"=w74:bool)  [unwired: 9 in]
  "Transform3d" <- w74
  n172 = call "report-test-results.vi"("error in (no error)"=w77, "TestPassed"=w74, "Test Name"="Transform3d") -> ("error out"=w75:errorcluster)  [unwired: 8 in]
  n173 = call "test-translation2d.vi"("error in (no error)"=w75) -> ("error out"=w161:errorcluster, "All PASSED"=w251:bool)  [unwired: 9 in]
  "Translation2d" <- w251
  n174 = call "report-test-results.vi"("error in (no error)"=w161, "TestPassed"=w251, "Test Name"="Translation2d") -> ("error out"=w85:errorcluster)  [unwired: 8 in]
  n175 = call "test-translation3d.vi"("error in (no error)"=w85) -> ("error out"=w87:errorcluster, "All PASSED"=w86:bool)  [unwired: 9 in]
  "Translation3d" <- w86
  n176 = call "report-test-results.vi"("error in (no error)"=w87, "TestPassed"=w86, "Test Name"="Translation3d") -> ("error out"=w84:errorcluster)  [unwired: 8 in]
  n177 = call "test-trapezoid-profile-ALL.vi"("error in (no error)"=w84) -> ("error out"=w162:errorcluster, "All TEsts passed"=w250:bool)  [unwired: 9 in]
  "Trapezoid Profile" <- w250
  n178 = call "report-test-results.vi"("error in (no error)"=w162, "TestPassed"=w250, "Test Name"="Trapezoid Profile") -> ("error out"=w153:errorcluster)  [unwired: 8 in]
  n179 = call "test-twist2d.vi"("error in (no error)"=w153) -> ("error out"=w163:errorcluster, "All PASSED"=w249:bool)  [unwired: 9 in]
  "Twist" <- w249
  n180 = call "report-test-results.vi"("error in (no error)"=w163, "TestPassed"=w249, "Test Name"="Twist2d") -> ("error out"=w90:errorcluster)  [unwired: 8 in]
  n181 = call "test-twist3d.vi"("error in (no error)"=w90) -> ("error out"=w92:errorcluster, "All PASSED"=w91:bool)  [unwired: 9 in]
  "Twist3d" <- w91
  n182 = call "report-test-results.vi"("error in (no error)"=w92, "TestPassed"=w91, "Test Name"="Twist3d") -> ("error out"=w89:errorcluster)  [unwired: 8 in]
  n183 = call "test-units.vi"("error in (no error)"=w89) -> ("error out"=w157:errorcluster, "All Tests Passed"=w248:bool)  [unwired: 9 in]
  "Units" <- w248
  n184 = call "report-test-results.vi"("error in (no error)"=w157, "TestPassed"=w248, "Test Name"="Units") -> ("error out"=w156:errorcluster)  [unwired: 8 in]
  n185 = call "test-unscented-kalman-filter-ALL.vi"("error in (no error)"=w156) -> ("error out"=w164:errorcluster, "All Tests Passed"=w246:bool)  [unwired: 9 in]
  "Unscented Kalman \nFilter" <- w246
  n186 = call "report-test-results.vi"("error in (no error)"=w164, "TestPassed"=w246, "Test Name"="Unscented Kalman Filter") -> ("error out"=w32:errorcluster)  [unwired: 8 in]
  n187 = call "test-vector-ALL-TESTS.vi"("error in (no error)"=w32) -> ("error out"=w34:errorcluster, "All Passed"=w33:bool)  [unwired: 9 in]
  "Vector" <- w33
  n188 = call "report-test-results.vi"("error in (no error)"=w34, "TestPassed"=w33, "Test Name"="Vector") -> ("error out"=w31:errorcluster)  [unwired: 8 in]
  n189 = call "test-Vision-Utils-ALL-TESTS.vi"("error in (no error)"=w31) -> ("error out"=w141:errorcluster, "All Passed"=w140:bool)  [unwired: 9 in]
  "Vision Utilities" <- w140
  n190 = call "report-test-results.vi"("error in (no error)"=w141, "TestPassed"=w140, "Test Name"="Vision Utilities") -> ("error out"=w17:errorcluster)  [unwired: 8 in]
  n191 = flat-sequence {
    tunnel: w17 -> [w369]
    frame #0 {
      n192 = call "report-test-completed.vi"("error in (no error)"=w369) -> ()  [unwired: 10 in, 1 out]
      "All Tests Finished" <- TRUE ("All Tests Finished")
    }
  }
